vi "RageATE_Send Email Attachment.vi"(0 "To: (email@site.com)":string="rickq@ragesystems.com", 1 "SMTP Outgoing Mail Server":string="smtp.office365.com", 2 "From: (email@site.com)":string="tomw@ragesystems.com", 5 "Subject:":string="LV SMTP", 7 "Body:":string="testing empty attachment path", 9 "Attachment Path":path, 11 "error in (no error)":errorcluster, 12 "Port":i32=587, 13 "Email Account ID":string="tomw@ragesystems.com", 14 "Email Account Password":string="175CabotSt!") -> (15 "error out":errorcluster)   [LabVIEW 2018]
panel:
  # "Overview: This example shows how to send email attachments from LabVIEW using any SMTP email service, such as Gmail.\nRequirements: LabVIEW 2012 (or compatible)\nInstructions: \n1. Configure all the controls on the front panel. If you use a Gmail account, set SMTP Outgping Mail Server to smtp.gmail.com\n2. Run the VI"
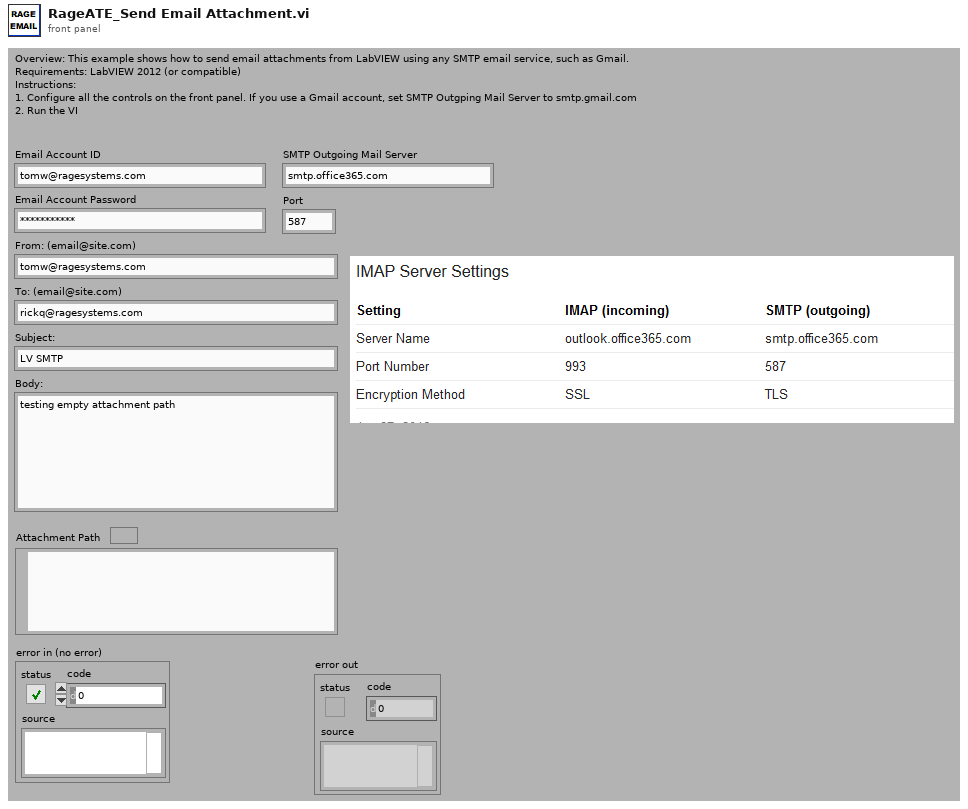
[diagram p1: front panel]
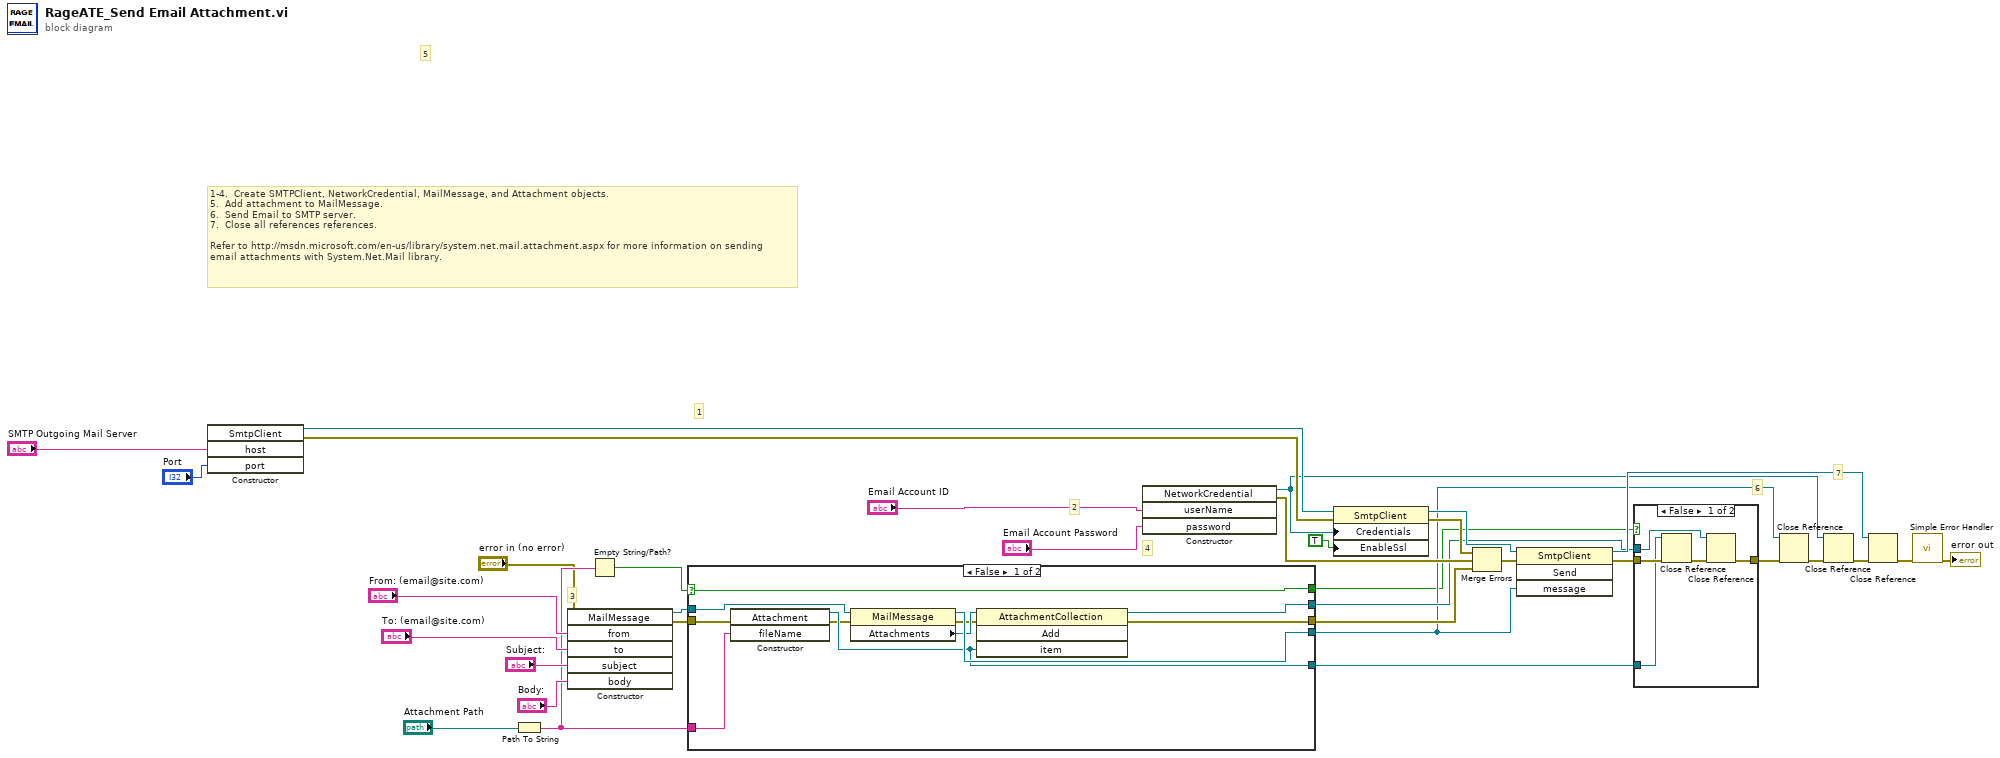
[diagram p0: block diagram]
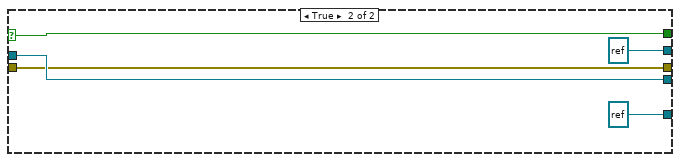
[diagram p3: hidden frame]
diagram:
  # "7"
  # "1-4.  Create SMTPClient, NetworkCredential, MailMessage, and Attachment objects.\n5.  Add attachment to MailMessage.\n6.  Send Email to SMTP server.\n7.  Close all references references.\n\nRefer to http://msdn.microsoft.com/en-us/library/system.net.mail.attachment.aspx for more information on sending\nemail attachments with System.Net.Mail library."
  # "6"
  # "5"
  # "4"
  # "3"
  # "2"
  # "1"
  n1 = constructor class="SmtpClient"("host"="SMTP Outgoing Mail Server", "port"="Port") -> (reference out=w34:refnum<k24>, error out=w21:errorcluster)  [unwired: 3 in, 3 out]
  n2 = Path To String(path="Attachment Path") -> (string=w6:string)
  n3 = constructor class="MailMessage"(error in="error in (no error)", "from"="From: (email@site.com)", "to"="To: (email@site.com)", "subject"="Subject:", "body"="Body:") -> (reference out=w22:refnum<k24>, error out=w7:errorcluster)  [unwired: 2 in, 5 out]
  n4 = Empty String/Path?(string/path=w6) -> (empty?=w4:bool)
  n5 = case shown="False" w4 {
    selector: w4 -> [w35 w46]
    tunnel: w22 -> [w45 w50]
    tunnel: [w44 w49] -> w16
    tunnel: [w43 refnum<k24> refnum ("Attachments")] -> w15
    tunnel: [w42 w50] -> w13
    tunnel: w7 -> [w41 w49]
    tunnel: w6 -> [w40 _]
    tunnel: [w39 refnum<k24> refnum ("new reference")] -> w5
    tunnel: [w35 w46] -> w3
    frame False {
      n6 = constructor class="Attachment"(error in=w41, "fileName"=w40) -> (reference out=w39:refnum<k24>, error out=w36:errorcluster)  [unwired: 2 in, 2 out]
      n7 = property class="MailMessage"(reference=w45, error in=w36) -> (reference out=w42:refnum<k24>, error out=w37:errorcluster, "Attachments"=w38:refnum<k24>)
      n8 = invoke class="AttachmentCollection" method="Add"(reference=w38, error in=w37, "item"=w39) -> (reference out=w43:refnum<k24>, error out=w44:errorcluster)  [unwired: 1 in, 2 out]
    }
    frame True {
    }
  }
  n9 = constructor class="NetworkCredential"("userName"="Email Account ID", "password"="Email Account Password") -> (reference out=w11:refnum<k24>, error out=w17:errorcluster)  [unwired: 3 in, 3 out]
  n10 = property class="SmtpClient"(reference=w34, error in=w21, "Credentials"=w11, "EnableSsl"=TRUE ("Enable SSL")) -> (reference out=w33:refnum<k24>, error out=w20:errorcluster)
  n11 = Merge Errors(w20, w17, w16) -> (w19:errorcluster)
  n12 = invoke class="SmtpClient" method="Send"(reference=w33, error in=w19, "message"=w13) -> (reference out=w18:refnum<k24>, error out=w8:errorcluster)  [unwired: 1 in, 2 out]
  n13 = case shown="False" w3 {
    tunnel: w15 -> [w55 _]
    tunnel: [w54 w56] -> w14
    tunnel: w8 -> [w53 w56]
    tunnel: w5 -> [w52 _]
    frame False {
      n14 = Close Reference(reference=w52, error in (no error)=w53) -> (error out=w51:errorcluster)
      n15 = Close Reference(reference=w55, error in (no error)=w51) -> (error out=w54:errorcluster)
    }
    frame True {
    }
  }
  n16 = Close Reference(reference=w13, error in (no error)=w14) -> (error out=w12:errorcluster)
  n17 = Close Reference(reference=w11, error in (no error)=w12) -> (error out=w10:errorcluster)
  n18 = Close Reference(reference=w18, error in (no error)=w10) -> (error out=w9:errorcluster)
  n19 = call <vilib>:"Simple Error Handler.vi"("error in (no error)"=w9) -> ("error out"=→"error out":errorcluster)  [unwired: 4 in, 4 out]
